vi "Format Summary String.vi"(8 "error in":errorcluster, 10 "FP":T1, 11 "Report":T2) -> (0 "error out":errorcluster, 1 "summary string header":string, 2 "summary string":string, 3 "full report string":string, 4 "Transition?":bool, 6 "Vac?":bool)   [LabVIEW 2018]
uses:
  Results.ctl
  Vacuum Test.ctl
  Vacuum Output.ctl
  Main Refs.ctl
  Hardware/Tecan/Pump Config.ctl
  Vacuum Specs.ctl
  Timing Specs.ctl
  Cartridges.ctl
  Cartridge Status.ctl
  Commands.ctl
  Lib/Time/Wells.ctl
  Lib/Time/Bottles.ctl
  Process State.ctl
panel:
  # "Tecan Pump"
  # "Vacuum"
  # "General"
  # "Timing"
  # "Protocol"
  # "Zaber"
  # "NFC Reader 1"
  # "NFC  Reader 2"
  # "NFC Reader 3"
  # "NFC Reader 4"
  # "System"
  # "Cartridge Utitlies"
  # "Wells"
  # "times"
  # "from"
  # "State Machine"
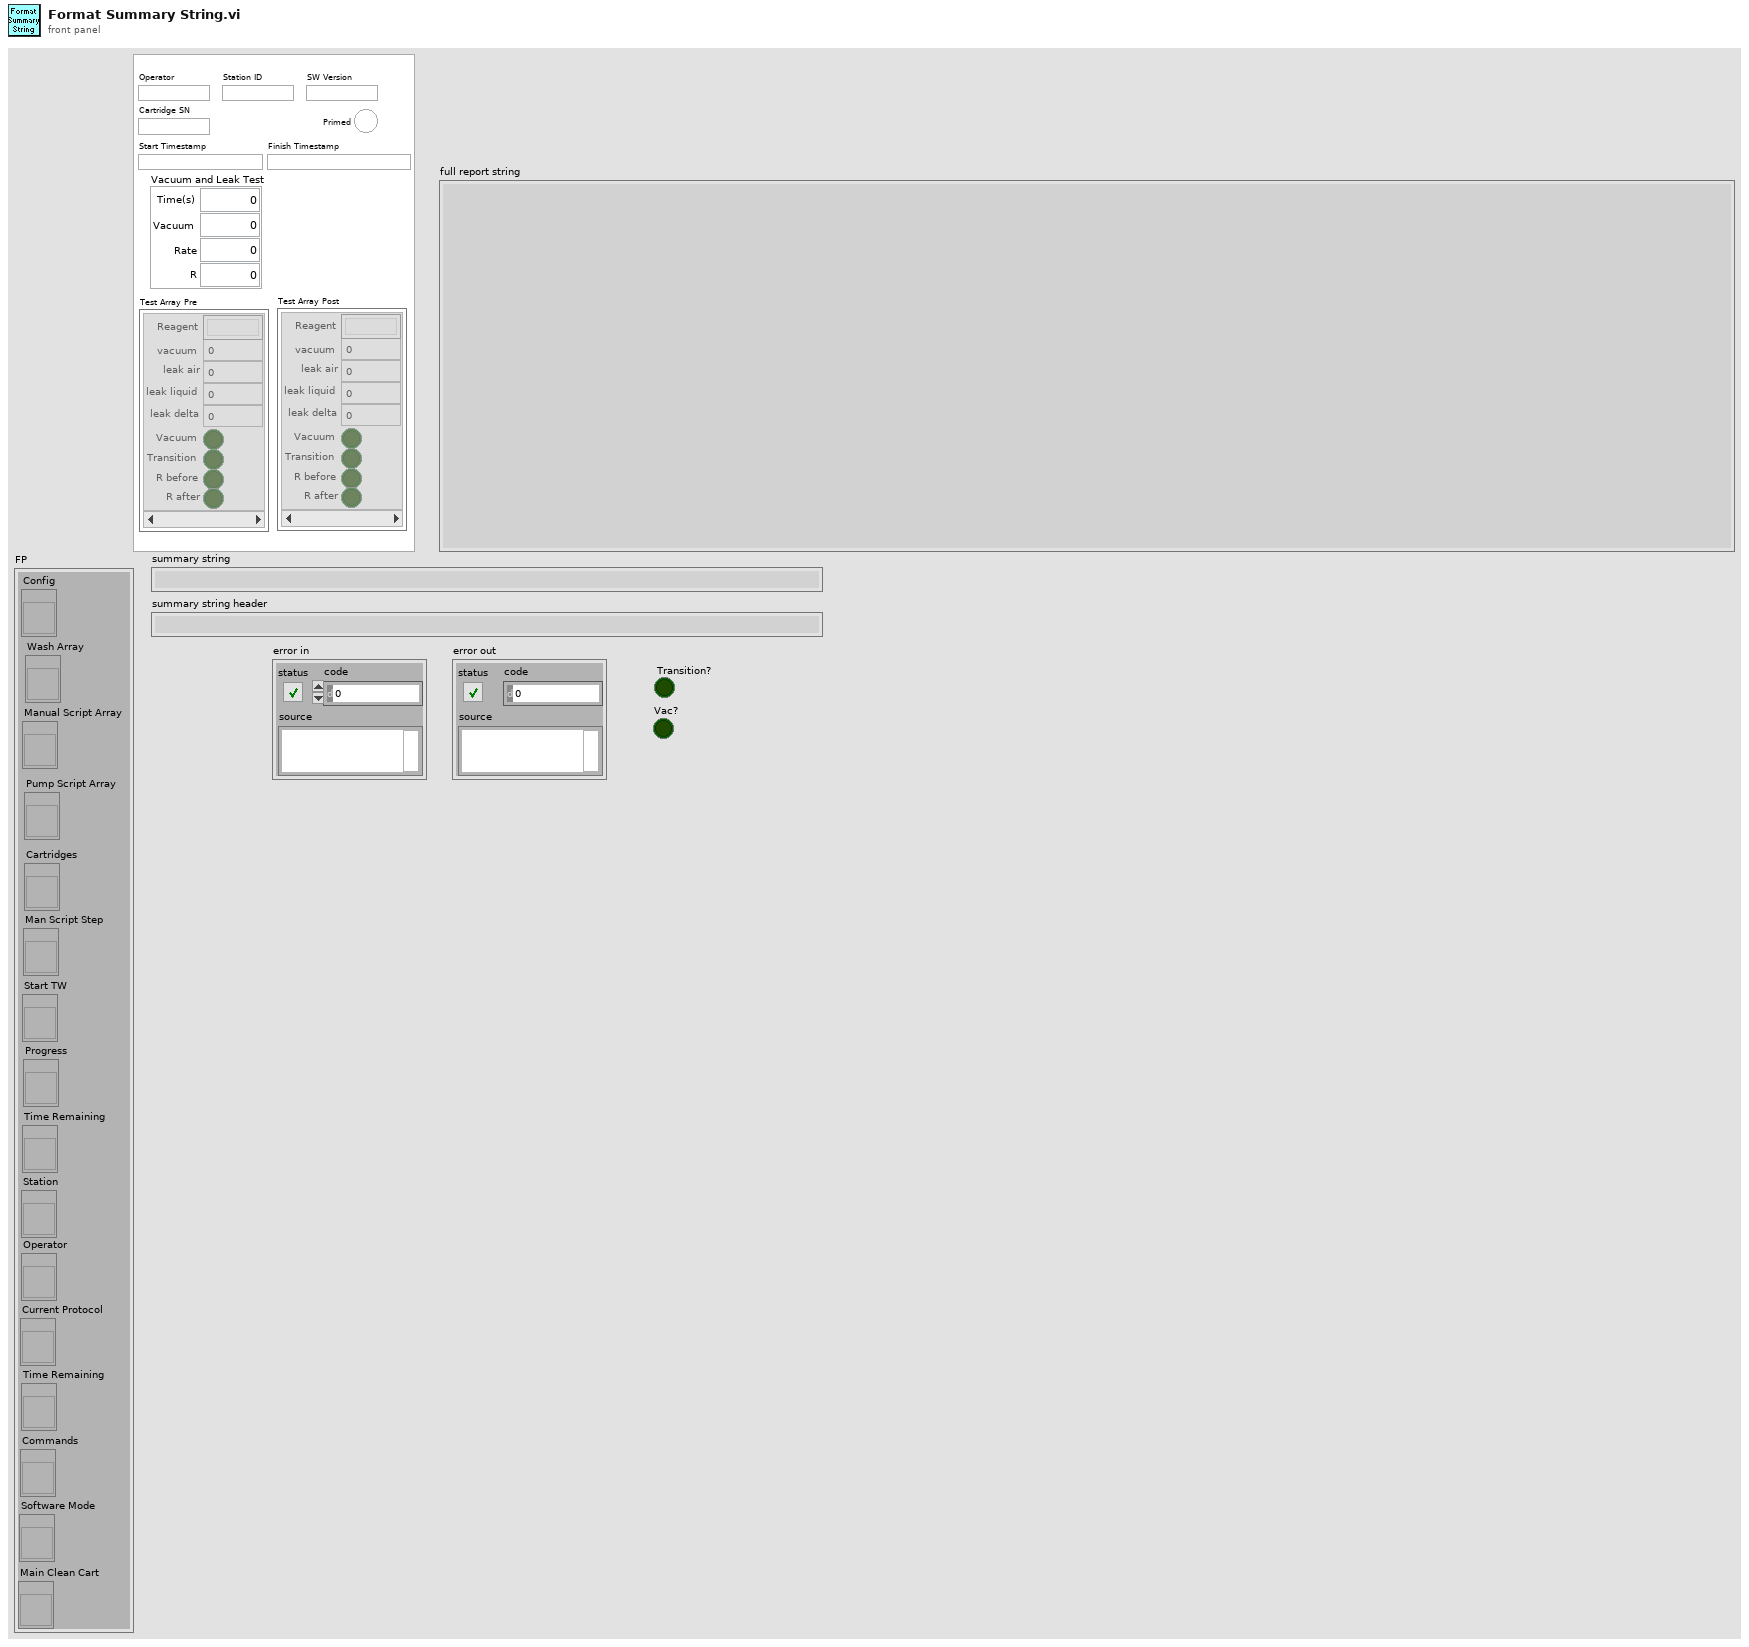
[diagram p1: front panel]
types:
  T1 = typedef "Main Refs.ctl" = cluster{"Config":refnum<vi>, "Wash Array":refnum<vi>, "Manual Script Array":refnum<vi>, "Pump Script Array":refnum<vi>, "Cartridges":refnum<vi>, "Man Script Step":refnum<vi>, "Start TW":refnum<vi>, "Progress":refnum<vi>, "Time Remaining":refnum<vi>, "Station":refnum<vi>, "Operator":refnum<vi>, "Current Protocol":refnum<vi>, "Time Remaining":refnum<vi>, "Commands":refnum<vi>, "Software Mode":refnum<vi>, "Main Clean Cart":refnum<vi>}
  T2 = typedef "Results.ctl" = cluster{"Operator":string, "Station ID":string, "SW Version":string, "Cartridge SN":string, "Primed":bool, "Start Timestamp":string, "Finish Timestamp":string, "Test Array Pre":T3[], "Test Array Post":T3[], "Vacuum and Leak Test":T4}
  T3 = typedef "Vacuum Test.ctl" = cluster{"vacuum":dbl, "leak air":dbl, "leak liquid":dbl, "leak delta":dbl, "Transition":bool, "Vacuum":bool, "R before":bool, "R after":bool, "Reagent":string}
  T4 = typedef "Vacuum Output.ctl" = cluster{"Time(s)":dbl, "Vacuum":dbl, "Rate":dbl, "R":dbl}
  T5 = typedef "Pump Config.ctl" = cluster{"Syringe size":u32, "Syringe address":u32, "# of ports":u32, "Init String":string, "Full Stroke (cnts)":i32, "Model":enum16{"XC", "Centris"}, "TW Position":dbl, "Load Position":dbl, "Bottom Position":dbl, "Station ID":string, "Vacuum Specs":T6, "Default Protocol":path, "Dry Time(s)":dbl, "Python Version":string, "NFC SN Array":string[], "Timing":T7}
  T6 = typedef "Vacuum Specs.ctl" = cluster{"vacuum max":dbl, "vacuum min":dbl, "liq2air rate delta":dbl, "liq2air time":dbl, "Conf. R":dbl, "LeakRateMax":dbl}
  T7 = typedef "Timing Specs.ctl" = cluster{"Checking vac and leak":dbl, "Priming input lines":dbl, "Rinsing syringe":dbl, "Filling well X w/ X":dbl, "Drain well X":dbl, "Clearing wells and lines":dbl, "Draining wells":dbl, "Rinsing all wells":dbl, "Testing for leaks/clogs":dbl, "Rinsing wells":dbl}
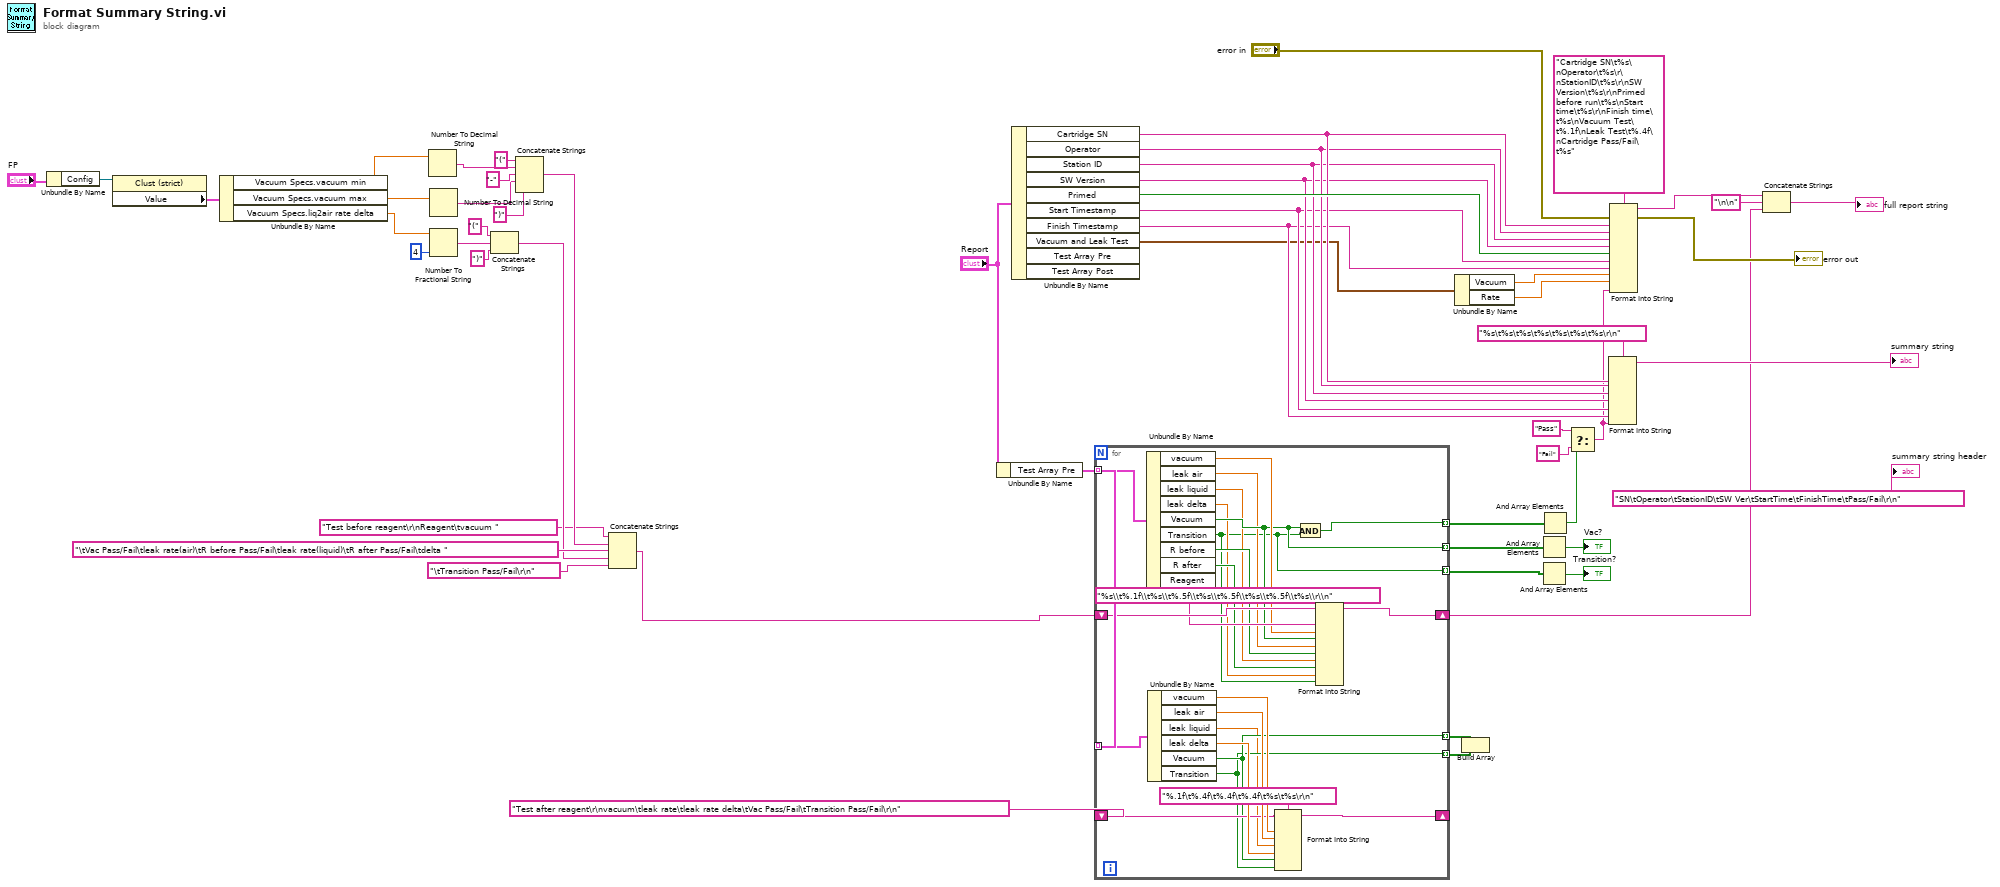
[diagram p0: block diagram]
diagram:
  n1 = Unbundle By Name("FP") -> ("Config"=w21:refnum<vi>)
  n2 = property class="Clust (strict)"(reference=w21) -> ("Value"=w20:T5)  [unwired: 1 in, 2 out]
  n3 = Unbundle By Name(w20) -> ("Vacuum Specs.vacuum min"=w19:dbl, "Vacuum Specs.vacuum max"=w18:dbl, "Vacuum Specs.liq2air rate delta"=w13:dbl)
  n4 = Number To Decimal String(number=w19) -> (decimal integer string=w17:string)  [unwired: 1 in]
  n5 = Number To Decimal String(number=w18) -> (decimal integer string=w15:string)  [unwired: 1 in]
  n6 = Number To Fractional String(number=w13, precision (6)=i16 4) -> (F-format string=w7:string)  [unwired: 2 in]
  n7 = Concatenate Strings("(" ("string"), w7, ")" ("string")) -> (w3:string)
  n8 = Concatenate Strings("(" ("string"), w17, "-" ("string"), w15, ")" ("string")) -> (w14:string)
  n9 = Concatenate Strings("Test before reagent\r\nReagent\tvacuum ", w14, "\tVac Pass/Fail\tleak rate(air)\tR before Pass/Fail\tleak rate(liquid)\tR after Pass/Fail\tdelta ", w3, "\tTransition Pass/Fail\r\n") -> (w11:string)
  n10 = Unbundle By Name("Report") -> ("Test Array Pre"=w30:T3[])
  n11 = Unbundle By Name("Report") -> ("Cartridge SN"=w50:string, "Operator"=w49:string, "Station ID"=w48:string, "SW Version"=w47:string, "Primed"=w51:bool, "Start Timestamp"=w46:string, "Finish Timestamp"=w42:string, "Vacuum and Leak Test"=w41:T4)  [unwired: 2 out]
  n12 = for {
    tunnel: w30 -> [w79] mode=indexing
    tunnel: w30 -> [w78] mode=indexing
    shift-right: [w72] -> w31
    shift-left: w11 -> [w71]
    shift-right: [w70] -> _
    shift-left: "Test after reagent\r\nvacuum\tleak rate\tleak rate delta\tVac Pass/Fail\tTransition Pass/Fail\r\n" -> [w69]
    tunnel: [w68] -> w35 mode=indexing
    tunnel: [w67] -> w34 mode=indexing
    tunnel: [w65] -> w28 mode=indexing
    tunnel: [w62] -> w26 mode=indexing
    tunnel: [w56] -> w23 mode=indexing
    n13 = Unbundle By Name(w79) -> ("vacuum"=w63:dbl, "leak air"=w61:dbl, "leak liquid"=w59:dbl, "leak delta"=w57:dbl, "Vacuum"=w62:bool, "Transition"=w56:bool, "R before"=w60:bool, "R after"=w58:bool, "Reagent"=w64:string)
    n14 = Unbundle By Name(w78) -> ("vacuum"=w77:dbl, "leak air"=w76:dbl, "leak liquid"=w66:dbl, "leak delta"=w75:dbl, "Vacuum"=w68:bool, "Transition"=w67:bool)
    n15 = Format Into String(format string="%.1f\t%.4f\t%.4f\t%.4f\t%s\t%s\r\n", initial string=w69, w77, w76, w66, w75, w68, w67) -> (resulting string=w70:string)  [unwired: 1 in, 1 out]
    n16 = And(x=w62, y=w56) -> (x .and. y?=w65:bool)
    n17 = Format Into String(format string="%s\\t%.1f\\t%s\\t%.5f\\t%s\\t%.5f\\t%s\\t%.5f\\t%s\\r\\n", initial string=w71, w64, w63, w62, w61, w60, w59, w58, w57, w56) -> (resulting string=w72:string)  [unwired: 1 in, 1 out]
  }
  n18 = Unbundle By Name(w41) -> ("Vacuum"=w40:dbl, "Rate"=w39:dbl)
  n19 = Build Array(w35, w34) -> ()  [unwired: 1 out]
  n20 = And Array Elements(Boolean array=w26) -> (logical AND=→"Vac?":bool)
  n21 = And Array Elements(Boolean array=w23) -> (logical AND=→"Transition?":bool)
  n22 = And Array Elements(Boolean array=w28) -> (logical AND=w27:bool)
  n23 = Select(t="Pass" ("Finish Timestamp"), s=w27, f="Fail" ("Finish Timestamp")) -> (s? t:f=w29:string)
  n24 = Format Into String(format string="%s\t%s\t%s\t%s\t%s\t%s\t%s\r\n", w50, w49, w48, w47, w46, w42, w29) -> (resulting string=→"summary string":string)  [unwired: 2 in, 1 out]
  n25 = Format Into String(format string="Cartridge SN\t%s\nOperator\t%s\r\nStationID\t%s\r\nSW Version\t%s\r\nPrimed before run\t%s\nStart time\t%s\r\nFinish time\t%s\nVacuum Test\t%.1f\nLeak Test\t%.4f\nCartridge Pass/Fail\t%s", error in="error in", w50, w49, w48, w47, w51, w46, w42, w40, w39, w29) -> (resulting string=w52:string, error out=→"error out":errorcluster)  [unwired: 1 in]
  n26 = Concatenate Strings(w52, "\n\n" ("string"), w31) -> (→"full report string":string)
  "summary string header" <- "SN\tOperator\tStationID\tSW Ver\tStartTime\tFinishTime\tPass/Fail\r\n" ("format string")
